vi "6c.vi"(11 "U":dbl) -> (3 "Array":dbl[](array[numeric]))   [LabVIEW 2016]
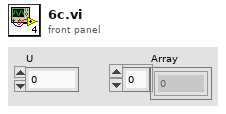
[diagram p1: front panel]
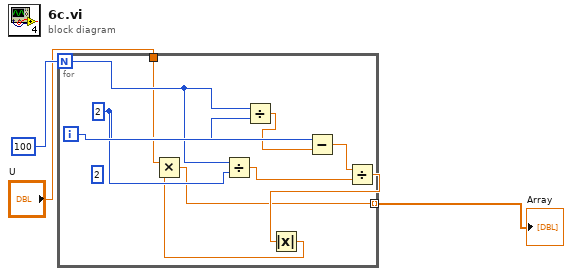
[diagram p0: block diagram]
diagram:
  n1 = for {
    N: 100 -> [w11]
    tunnel: "U" -> [w6]
    tunnel: [w4] -> w2 mode=indexing
    i -> [w13]
    (unwired) 2
    w10 = 2
    n2 = Divide(x=w11, y=w10) -> (x/y=w8:dbl)
    n3 = Divide(x=w11, y=w10) -> (x/y=w12:dbl)
    n4 = Subtract(x=w13, y=w12) -> (x-y=w9:dbl)
    n5 = Divide(x=w9, y=w8) -> (x/y=w7:dbl)
    n6 = Absolute Value(x=w7) -> (abs(x)=w5:dbl)
    n7 = Multiply(x=w6, y=w5) -> (x*y=w4:dbl)
  }
  "Array" <- w2
